vi "Set UUT Serial Port Parameters.vi"(0 "VISA resource name":refnum<visa-resource-name>, 1 "Baud Rate (9600)":u32=9600, 5 "Flow Control (0: Xon/Xoff)":u32(ring) items=["Xon/Xoff", "None", "Rts/Cts"], 7 "Number Data Bits (1: 8 bits)":u32(ring)=1 items=["7 bits", "8 bits"], 9 "Number Stop Bits (0: 1 bit)":u32(ring) items=["1 bit", "2 bits"], 11 "error in (no error)":errorcluster, 12 "Parity  (0: None)":u32(ring) items=["None", "Odd", "Even"]) -> (4 "VISA resource name out":refnum<visa-resource-name>, 15 "error out":errorcluster)   [LabVIEW 2013, in "Fluke 5XXX Series Multicalibrators.lvlib"]
doc: "This VI Sets the RS-232-C settings for the Calibrator rear panel SERIAL 2 TO UUT serial port, which is saved in the Calibrator non-volatile memory. (While saving configuration data in the non-volatile memory, a period of about 2 seconds, the Calibrator does not respond to remote commands.)\n\nNote:\n\nThis VI is available only for instrument models 5500A and 5520A."
uses:
  Fluke 5XXX Series Multicalibrators.lvlib
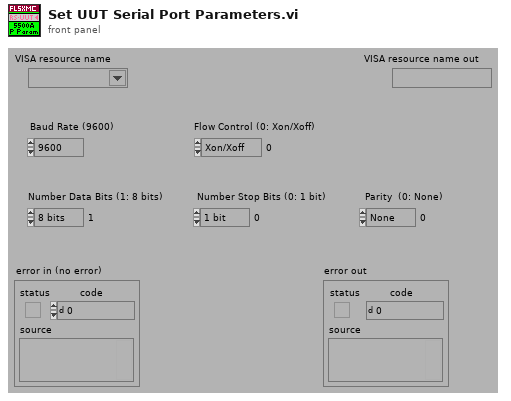
[diagram p1: front panel]
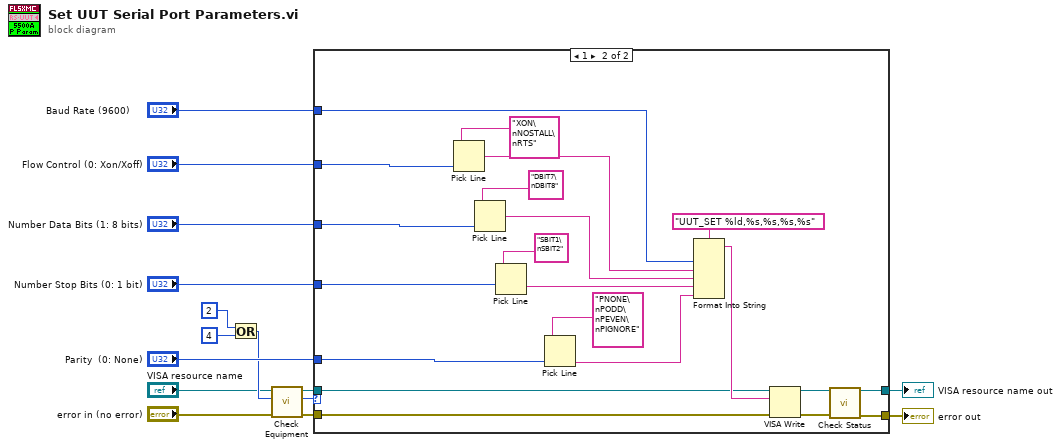
[diagram p0: block diagram]
diagram:
  n1 = Or(x=2 ("Numeric"), y=4 ("Numeric")) -> (x .or. y?=w6:i32)
  n2 = call "Check Equipment.vi"("error in (no error)"="error in (no error)", "Bit Mask"=w6, "VISA resource name"="VISA resource name") -> ("error out"=w1:errorcluster, "Present?"=w2:u32, "VISA resource name out"=w3:refnum<visa-resource-name>)  [unwired: 6 in]
  n3 = case shown="1" w2 {
    tunnel: "Baud Rate (9600)" -> [_ w19]
    tunnel: [w16 w29] -> w14
    tunnel: w3 -> [w17 w28]
    tunnel: "Flow Control (0: Xon/Xoff)" -> [_ w27]
    tunnel: "Number Data Bits (1: 8 bits)" -> [_ w26]
    tunnel: "Number Stop Bits (0: 1 bit)" -> [_ w25]
    tunnel: "Parity  (0: None)" -> [_ w24]
    tunnel: [w17 w20] -> w9
    tunnel: w1 -> [w16 w18]
    frame 0, Default {
    }
    frame 1 {
      n4 = Pick Line(multi-line string="XON\nNOSTALL\nRTS" ("Reset Command"), line index=w27) -> (output string=w34:string)  [unwired: 1 in]
      n5 = Pick Line(multi-line string="DBIT7\nDBIT8" ("Reset Command"), line index=w26) -> (output string=w21:string)  [unwired: 1 in]
      n6 = Pick Line(multi-line string="SBIT1\nSBIT2" ("Reset Command"), line index=w25) -> (output string=w22:string)  [unwired: 1 in]
      n7 = Pick Line(multi-line string="PNONE\nPODD\nPEVEN\nPIGNORE" ("Reset Command"), line index=w24) -> (output string=w23:string)  [unwired: 1 in]
      n8 = Format Into String(format string="UUT_SET %ld,%s,%s,%s,%s" ("Reset Command"), w19, w34, w21, w22, w23) -> (resulting string=w35:string)  [unwired: 2 in, 1 out]
      n9 = VISA Write(VISA resource name=w28, write buffer=w35, error in (no error)=w18) -> (VISA resource name out=w38:refnum<visa-resource-name>, error out=w37:errorcluster)  [unwired: 1 out]
      n10 = call "Check Status.vi"("VISA resource name"=w38, "error in (no error)"=w37) -> ("VISA resource name out"=w20:refnum<visa-resource-name>, "error out"=w29:errorcluster)  [unwired: 12 in]
    }
  }
  "VISA resource name out" <- w9
  "error out" <- w14
